vi "Actor Core.vi"(8 "error in":errorcluster, 11 "Nested in":refnum<class "UI_Top_Customer.lvclass">) -> (0 "error out":errorcluster, 3 "Actor out":refnum<class "Actor.lvclass">)   [LabVIEW 2021, in "UI_Top_Customer.lvclass"]
doc: "(<B>Filename</B>: Actor Framework.lvlib:Actor.lvclass:Actor Core.vi)\n\nReceives messages to the actor, reacts to them, and initiates any error handling that may shut the actor down.\n\nDescendant classes may override this VI to append parallel tasks for the actor to complete while it handles messages. Overrides use the Call Parent Method node."
uses:
  UI_Top_Customer.lvclass
  <vilib>/ActorFramework/Actor/Actor.lvclass
  <vilib>/ActorFramework/Stop Msg/Stop Msg.lvclass
  <userlib>/John_Lib/AbstractActorTemplate/AbstractActorTemplate/UIActorTop.lvclass
  <userlib>/John_Lib/AbstractActorTemplate/UIActorTop Messages/UI Front Panel State Msg/UI Front Panel State Msg.lvclass
  <userlib>/John_Lib/Control/Panel State.ctl
  <vilib>/Utility/miscctls.llb/LVRectTypeDef.ctl
  <userlib>/John_Lib/Queue_Self/Queue_Self.lvlib
  C:/Program Files (x86)/National Instruments/LabVIEW 2021/vi.lib/ActorFramework/Actor/Actor.lvclass
  C:/Program Files (x86)/National Instruments/LabVIEW 2021/user.lib/John_Lib/AbstractActorTemplate/AbstractActorTemplate/UIActorTop.lvclass
  Launcher/Min Button.ctl
  Buttons.ctl
panel:
  out "B_UpSide":bool
  in  "Button":T1
  out "B_RightSide":bool
  out "B_DownSide":bool
  out "B_LeftSide":bool
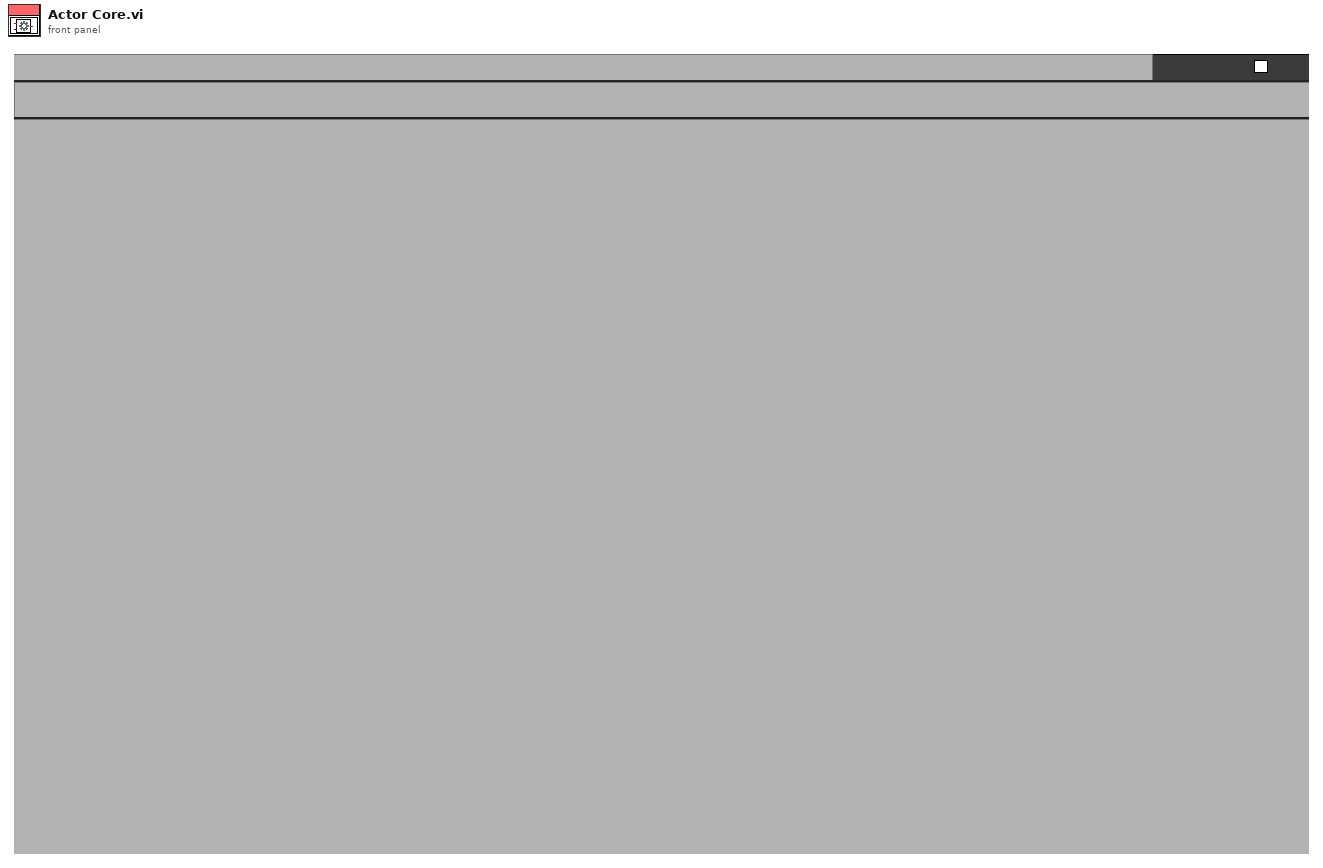
[diagram p1: front panel]
types:
  T1 = typedef "UI_Top_Customer.lvclass/Buttons.ctl" = cluster{"Min Button":T2, "Max Button":bool, "Cancel Button":bool}
  T2 = typedef "UI_Top_Customer.lvclass/Min Button.ctl" = bool
  T3 = typedef "LVRectTypeDef.ctl" = cluster{"Left":i16, "Top":i16, "Right":i16, "Bottom":i16}
  T4 = enum32{"Invalid", "Standard", "Closed", "Hidden", "Minimized", "Maximized"}
  T5 = typedef "Panel State.ctl" = string
  T6 = typedef "LVPoint32TypeDef.ctl" = cluster{"Horizontal":i32, "Vertical":i32}
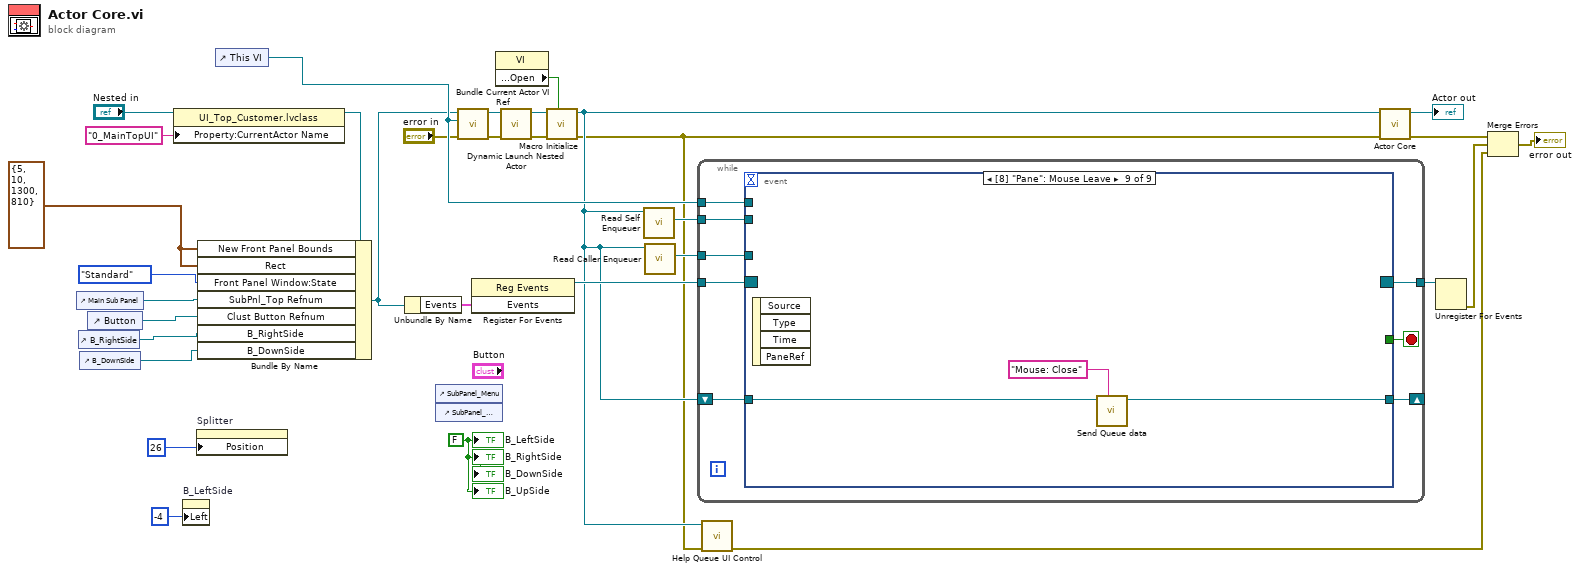
[diagram p0: block diagram]
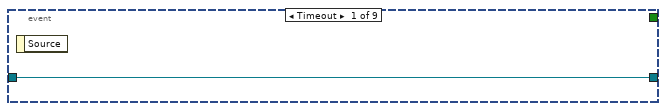
[diagram p2: hidden frame]
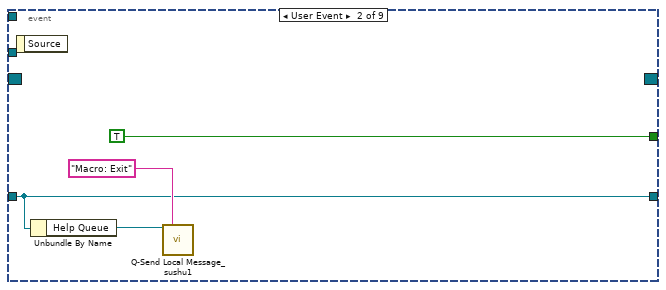
[diagram p3: hidden frame]
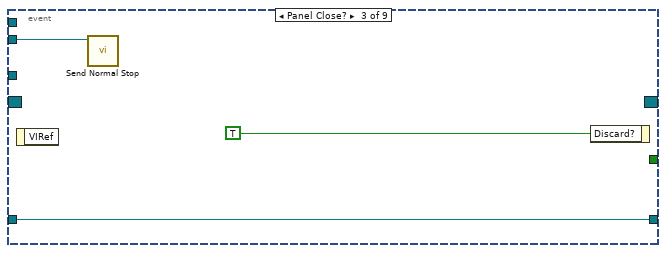
[diagram p4: hidden frame]
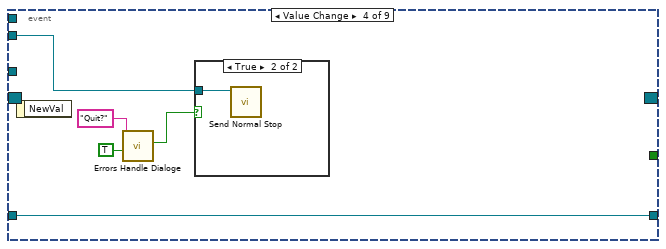
[diagram p5: hidden frame]
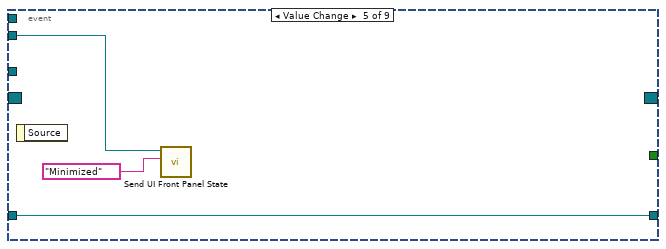
[diagram p7: hidden frame]
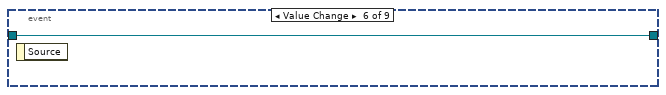
[diagram p8: hidden frame]
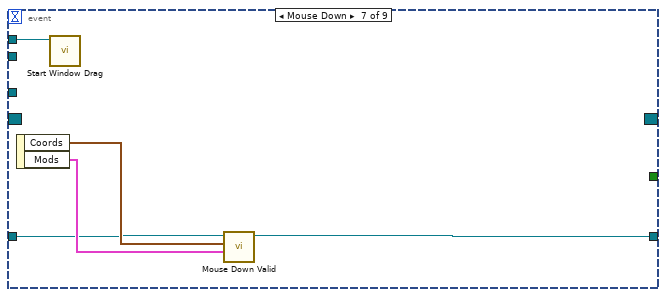
[diagram p9: hidden frame]
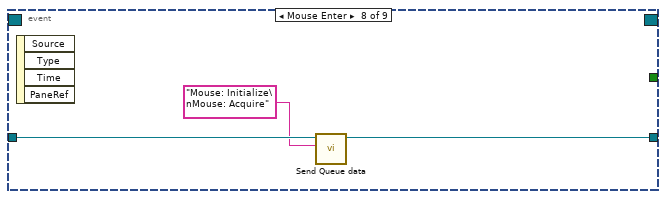
[diagram p10: hidden frame]
diagram:
  w9 = FALSE ("B_LeftSide")
  w11 = T3 {"Left"=5, "Top"=10, "Right"=1300, "Bottom"=810} ("Front Panel Window:Panel Bounds")
  n1 = control-ref of="Main Sub Panel"() -> (w18:refnum<vi>)
  n2 = control-ref of="B_RightSide"() -> (w14:refnum<vi>)
  n3 = control-ref of="B_DownSide"() -> (w13:refnum<vi>)
  n4 = control-ref of="Button"() -> (w17:refnum<vi>)
  n5 = property class="UI_Top_Customer.lvclass"(reference="Nested in", "Property:CurrentActor Name"="0_MainTopUI" ("AbstractActor:CurrentActor Name")) -> (reference out=w7:refnum<class "UI_Top_Customer.lvclass">)  [unwired: 1 in, 1 out]
  n6 = property on="B_LeftSide" class="Bool (strict)"("Left"=-4 ("Position:Left")) -> ()  [unwired: 2 in, 2 out]
  n7 = property on="Splitter" class="Splitter"("Position"=26 ("Splitter Position 2")) -> ()  [unwired: 2 in, 2 out]
  n8 = Bundle By Name(cluster=w7, "New Front Panel Bounds"=w11, "Rect"=w11, "Front Panel Window:State"=T4."Standard", "SubPnl_Top Refnum"=w18, "Clust Button Refnum"=w17, "B_RightSide"=w14, "B_DownSide"=w13) -> (w6:refnum<class "UI_Top_Customer.lvclass">)
  n9 = control-ref of="This VI"() -> (w12:refnum<vi>)
  n10 = Unbundle By Name(w6) -> ("Events"=w30:cluster{"Stop":refnum<user-event>})
  n11 = control-ref of="SubPanel_Menu"() -> ()  [unwired: 1 out]
  n12 = control-ref of="SubPanel_Button"() -> ()  [unwired: 1 out]
  n13 = call <userlib>:"Bundle Current Actor VI Ref.vi"("error in (no error)"="error in", "This VI"=w12, "UI ActorTop in"=w6) -> ("error out"=w19:errorcluster, "UI ActorTop out"=w20:refnum<class "UI_Top_Customer.lvclass">)  [unwired: 5 in, 2 out]
  n14 = register-events ("Main Register for Events")(w30) -> (reference out=w31:refnum<event-registration>)  [unwired: 2 in, 1 out]
  n15 = property class="VI"() -> ("Front Panel.Open"=w26:bool)  [unwired: 2 in, 2 out]
  n16 = call-dynamic "Dynamic Launch Nested Actor.vi"("error in (no error)"=w19, "UI ActorTop in"=w20) -> ("error out"=w27:errorcluster, "UI ActorTop out"=w28:refnum<class "UI_Top_Customer.lvclass">)  [unwired: 8 in]
  n17 = call-dynamic "Macro Initialize.vi"("Front Panel Window:Open"=w26, "error in (no error)"=w27, "UI ActorTop in"=w28) -> ("error out"=w1:errorcluster, "UI ActorTop out"=w8:refnum<class "UI_Top_Customer.lvclass">)  [unwired: 7 in]
  n18 = call <vilib>:"Read Self Enqueuer.vi"("Actor"=w8) -> ("Self Enqueuer"=w10:refnum<class "Message Enqueuer.lvclass">)  [unwired: 10 in]
  n19 = call <vilib>:"Read Caller Enqueuer.vi"("Actor"=w8) -> ("Caller Enqueuer"=w22:refnum<class "Message Enqueuer.lvclass">)  [unwired: 10 in]
  n20 = while {
    tunnel: w31 -> [w40]
    tunnel: [w38] -> w29
    tunnel: w10 -> [w37]
    tunnel: w22 -> [w36]
    tunnel: w12 -> [w35]
    shift-right: [w33] -> _
    shift-left: w8 -> [w34]
    stop <- w39 stop-if-true
    n21 = event "UI Events" shown="[8] \"Pane\": Mouse Leave" {
      selector: w40 -> [_ _ _ _ _ _ _ _ _]
      dyn-events: [_ _ _ _ _ _ _ _ _] -> w38
      timeout: _ -> [_ _ _ _ _ _ _ _ _]
      tunnel: [_ TRUE _ _ _ _ _ _ _] -> w39
      tunnel: w37 -> [_ _ w47 w53 w57 _ _ _ _]
      tunnel: w36 -> [_ _ _ _ _ _ _ _ _]
      tunnel: w35 -> [_ _ _ _ _ _ w63 _ _]
      tunnel: w34 -> [w41 w43 w46 w49 w55 w58 w59 w65 w68]
      tunnel: [w41 w43 w46 w49 w55 w58 w60 w66 w69] -> w33
      event Timeout {
        n22 = event-data() -> ()  [unwired: 1 in, 1 out]
      }
      event User Event {
        n23 = event-data() -> ()  [unwired: 1 in, 1 out]
        n24 = Unbundle By Name(w43) -> ("Help Queue"=w42:refnum<queue>)
        n25 = call <userlib>:"Q-Send Local Message_sushu1.vi"("queue in"=w42, "Elements in Front"="Macro: Exit") -> ()  [unwired: 11 in, 3 out]
      }
      event Panel Close? {
        n26 = event-data() -> ()  [unwired: 1 in, 1 out]
        n27 = call <vilib>:"Send Normal Stop.vi"("Message Enqueuer"=w47) -> ()  [unwired: 10 in, 1 out]
        n28 = event-data("Discard?"=TRUE) -> ()  [unwired: 1 in, 1 out]
      }
      event Value Change {
        n29 = event-data() -> ()  [unwired: 1 in, 1 out]
        n30 = call <userlib>:"Errors Handle Dialoge.vi"("DisplayDialog"=TRUE, "Message"="Quit?") -> ("OK?"=w50:bool)  [unwired: 8 in, 1 out]
        n31 = case shown="True" w50 {
          tunnel: w53 -> [_ w54]
          frame False {
          }
          frame True {
            n32 = call <vilib>:"Send Normal Stop.vi"("Message Enqueuer"=w54) -> ()  [unwired: 10 in, 1 out]
          }
        }
      }
      event Value Change {
        n33 = event-data() -> ()  [unwired: 1 in, 1 out]
        n34 = call <userlib>:"Send UI Front Panel State.vi"("Argument"=T5 "Minimized", "Message Enqueuer"=w57) -> ()  [unwired: 8 in, 2 out]
      }
      event Value Change {
        n35 = event-data() -> ()  [unwired: 1 in, 1 out]
      }
      event Mouse Down {
        n36 = event-data() -> ("Coords"=w62:T6, "Mods"=w61:cluster{"Double Click":bool, "Menu Key":bool})  [unwired: 1 in]
        n37 = call <userlib>:"Start Window Drag.vi"("VI Ref (calling VI)"=w63) -> ()  [unwired: 9 in, 2 out]
        n38 = call "Mouse Down Valid.vi"("Mods"=w61, "Coords"=w62, "UI_Top_Customer in"=w59) -> ("UI_Top_Customer out"=w60:refnum<class "UI_Top_Customer.lvclass">)  [unwired: 7 in, 1 out]
      }
      event Mouse Enter {
        n39 = event-data() -> ()  [unwired: 1 in, 4 out]
        n40 = call "Send Queue data.vi"("Elements at Back"="Mouse: Initialize\nMouse: Acquire", "UI_Top_Customer in"=w65) -> ("UI_Top_Customer out"=w66:refnum<class "UI_Top_Customer.lvclass">)  [unwired: 8 in, 1 out]
      }
      event Mouse Leave {
        n41 = event-data() -> ()  [unwired: 1 in, 4 out]
        n42 = call "Send Queue data.vi"("Elements in Front"="Mouse: Close", "UI_Top_Customer in"=w68) -> ("UI_Top_Customer out"=w69:refnum<class "UI_Top_Customer.lvclass">)  [unwired: 8 in, 1 out]
      }
    }
  }
  n43 = call "Help Queue UI Control.vi"("error In"=w1, "UI_Top_Customer in"=w8) -> ("error out"=w2:errorcluster)  [unwired: 9 in]
  n44 = call-parent "Actor Core.vi"("error in"=w1, "Actor in"=w8) -> ("error out"=w24:errorcluster, "Actor out"=→"Actor out":refnum<class "Actor.lvclass">)  [unwired: 8 in]
  n45 = Unregister For Events(event registration refnum=w29) -> (error out=w25:errorcluster)  [unwired: 1 in]
  n46 = Merge Errors(w24, w25, w2) -> (→"error out":errorcluster)
  "B_LeftSide" <- w9
  "B_DownSide" <- w9
  "B_RightSide" <- w9
  "B_UpSide" <- w9
